vi "sub_ch-count.vi"(11 "ch config":bool[](array[boolean])) -> (3 "ch num":u8)   [LabVIEW 2019]
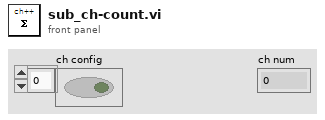
[diagram p1: front panel]
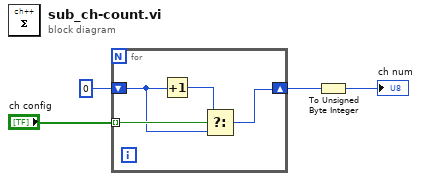
[diagram p0: block diagram]
diagram:
  n1 = for {
    tunnel: "ch config" -> [w8] mode=indexing
    shift-right: [w5] -> w4
    shift-left: 0 -> [w6]
    n2 = Increment(x=w6) -> (x+1=w7:i32)
    n3 = Select(t=w7, s=w8, f=w6) -> (s? t:f=w5:i32)
  }
  n4 = To Unsigned Byte Integer(number=w4) -> (unsigned 8bit integer=→"ch num":u8)
